vi "Rename Links.vi"(8 "error in (no error)":errorcluster, 9 "New Name":string, 10 "Old Name":string, 11 "State in":refnum<class "State.lvclass">) -> (0 "error out":errorcluster, 3 "State out":refnum<class "State.lvclass">)   [LabVIEW 2015, in "State.lvclass"]
uses:
  State.lvclass
  State.lvclass/State.ctl
  Termination/Termination.lvclass
  Timeout/Timeout.lvclass
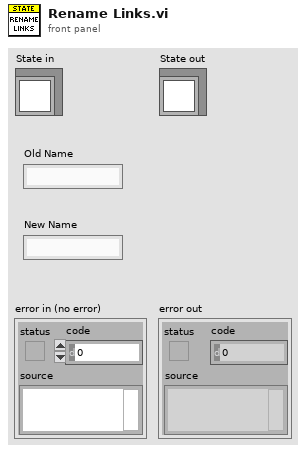
[diagram p1: front panel]
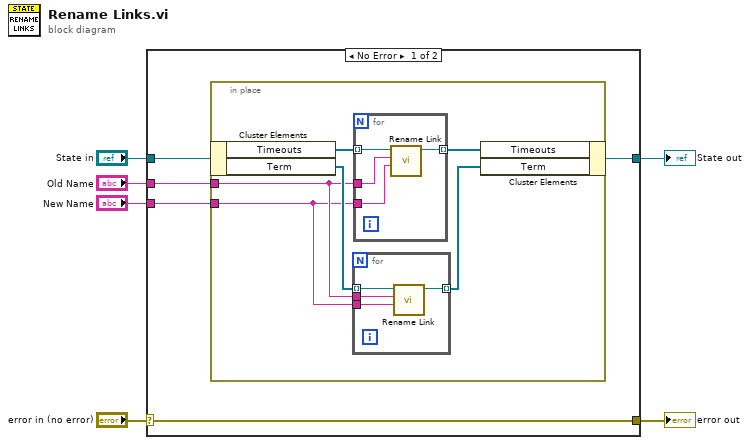
[diagram p0: block diagram]
diagram:
  n1 = case shown="No Error" "error in (no error)" {
    selector: "error in (no error)" -> [w11 w27]
    tunnel: [w11 w27] -> w5
    tunnel: [w9 w26] -> w3
    tunnel: "State in" -> [w10 w26]
    tunnel: "Old Name" -> [w8 _]
    tunnel: "New Name" -> [w7 _]
    frame No Error {
      n2 = in-place {
        in-place-border: w8 -> [w13]
        in-place-border: w7 -> [w12]
        n3 = in-place-cluster #1(w10) -> ("Timeouts"=w17:refnum<class "Timeout.lvclass">[], "Term"=w15:refnum<class "Termination.lvclass">[])
        n4 = for {
          tunnel: w15 -> [w21] mode=indexing
          tunnel: [w18] -> w14 mode=indexing
          tunnel: w13 -> [w20]
          tunnel: w12 -> [w19]
          n5 = call "Rename Link.vi"("New Name"=w19, "Old Name"=w20, "Termination in"=w21) -> ("Termination out"=w18:refnum<class "Termination.lvclass">)  [unwired: 7 in, 1 out]
        }
        n6 = for {
          tunnel: w17 -> [w25] mode=indexing
          tunnel: [w22] -> w16 mode=indexing
          tunnel: w13 -> [w24]
          tunnel: w12 -> [w23]
          n7 = call "Rename Link.vi"("New Name"=w23, "Old Name"=w24, "Timeout in"=w25) -> ("Timeout out"=w22:refnum<class "Timeout.lvclass">)  [unwired: 7 in, 1 out]
        }
        n8 = in-place-cluster #1("Timeouts"=w16, "Term"=w14) -> (w9:refnum<class "State.lvclass">)
      }
    }
    frame Error {
    }
  }
  "error out" <- w5
  "State out" <- w3
